vi "load_panel.vi"() -> ()   [LabVIEW 2013]
uses:
  RydbergExpControl/red_mot_controls.ctl
panel:
  out "Tree":string(tree)
  in  "XML File Path":path
  in  "Inputs":T1 {"Waveform Parameters"."Degree" min=1}
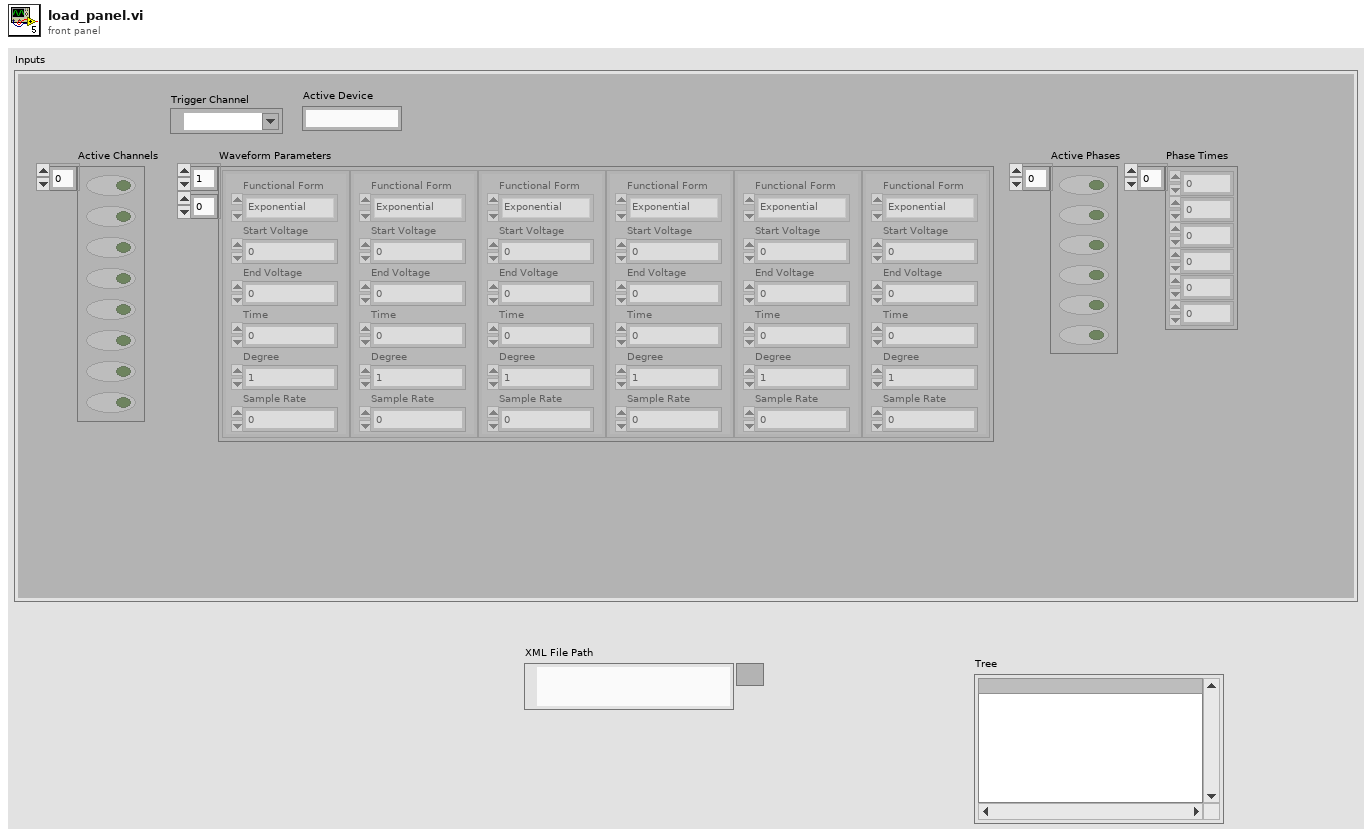
[diagram p1: front panel]
types:
  T1 = typedef "red_mot_controls.ctl" = cluster{"Active Device":string, "Active Channels":bool[], "Waveform Parameters":cluster{"Functional Form":enum16{"Polynomial", "Exponential"}, "Start Voltage":dbl, "End Voltage":dbl, "Time":dbl, "Degree":i8, "Sample Rate":dbl}[][], "Active Phases":bool[], "Phase Times":dbl[], "Trigger Channel":tag}
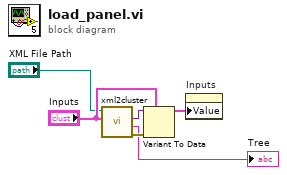
[diagram p0: block diagram]
diagram:
  n1 = call "xml2cluster.vi"("TypeDesc"="Inputs", "XML File Path"="XML File Path") -> ("error out"=w3:errorcluster, "XML String Out"=→"Tree":string, "data"=w6:variant)  [unwired: 7 in]
  n2 = Variant To Data(error in=w3, type="Inputs", Variant=w6) -> (data=w2:T1)  [unwired: 1 out]
  n3 = property on="Inputs" class="Clust (strict)"("Value"=w2) -> ()  [unwired: 2 in, 2 out]
